vi "GetControlTerminals.vi"(6 "error in":errorcluster, 9 "VI Interpreter in":refnum<class "VI Interpreter.lvclass">) -> (0 "error out":errorcluster, 3 "VI Interpreter out":refnum<class "VI Interpreter.lvclass">, 4 "controls":refnum<class "ControlTerminal.lvclass">[](array[class]))   [LabVIEW 2014, in "Raspberry Pi Compatible Compiler for LabVIEW.lvlib" / "VI Interpreter.lvclass"]
uses:
  VI Interpreter.lvclass
  ControlTerminal/ControlTerminal.lvclass
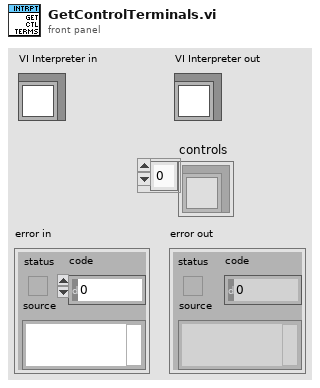
[diagram p1: front panel]
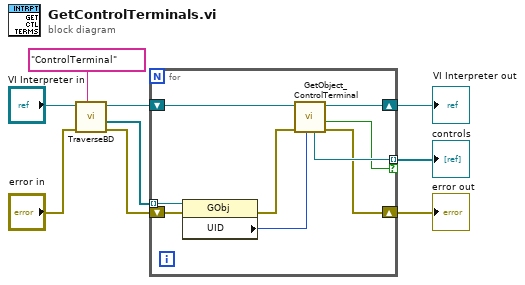
[diagram p0: block diagram]
diagram:
  n1 = call "TraverseBD.vi"("class name"="ControlTerminal", "error in"="error in", "VI Interpreter in"="VI Interpreter in") -> ("error out"=w4:errorcluster, "References"=w2:refnum<vi>[], "VI Interpreter out"=w5:refnum<class "VI Interpreter.lvclass">)  [unwired: 4 in]
  n2 = for {
    tunnel: w2 -> [w13] mode=indexing
    shift-right: [w17] -> w9
    shift-left: w5 -> [w18]
    tunnel: [w16] -> w7 mode=indexing if=w15
    shift-right: [w14] -> w8
    shift-left: w4 -> [w12]
    n3 = property class="GObj"(reference=w13, error in=w12) -> (error out=w10:errorcluster, "UID"=w11:i32)  [unwired: 1 out]
    n4 = call "GetObject_ControlTerminal.vi"("UID"=w11, "error in"=w10, "VI Interpreter in"=w18) -> ("error out"=w14:errorcluster, "found"=w15:bool, "VI Interpreter out"=w17:refnum<class "VI Interpreter.lvclass">, "control"=w16:refnum<class "ControlTerminal.lvclass">)  [unwired: 3 in]
  }
  "error out" <- w8
  "VI Interpreter out" <- w9
  "controls" <- w7
